vi "Label Printing.vi"(6 "Print?":bool, 7 "PN":string, 8 "error in (no error)":errorcluster, 9 "SN":string, 10 "DT":string, 11 "Path":path=path "D:/Valeo/Micriphone Test/UI/ME79.btw") -> (0 "error out":errorcluster)   [LabVIEW 2018]
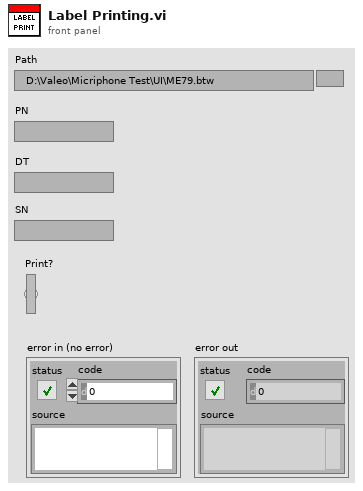
[diagram p1: front panel]
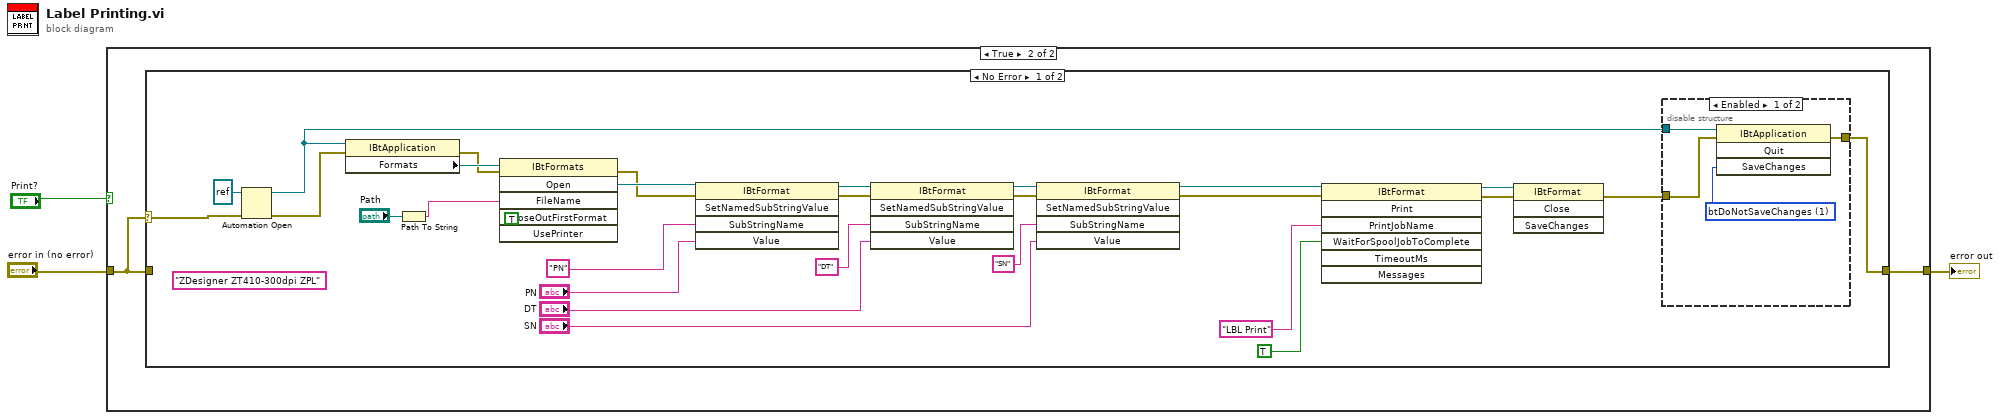
[diagram p0: block diagram]
diagram:
  n1 = case shown="True" "Print?" {
    tunnel: "error in (no error)" -> [w4 w5]
    tunnel: [w4 w6] -> w1
    frame False {
    }
    frame True {
      n2 = case shown="No Error" w5 {
        selector: w5 -> [w26 _]
        tunnel: [w27 w40] -> w6
        tunnel: w5 -> [_ w40]
        frame No Error {
          (unwired) "ZDesigner ZT410-300dpi ZPL" ("UsePrinter")
          (unwired) TRUE ("CloseOutFirstFormat")
          n3 = Automation Open(error in (no error)=w26, Automation Refnum=refnum<k7> refnum ("BarTender.IBtApplication")) -> (Automation Refnum=w13:refnum<k7>, error out=w12:errorcluster)  [unwired: 2 in]
          n4 = property class="IBtApplication"(reference=w13, error in=w12) -> (error out=w8:errorcluster, "Formats"=w11:refnum<k7>)  [unwired: 1 out]
          n5 = Path To String(path="Path") -> (string=w9:string)
          n6 = invoke class="IBtFormats" method="Open"(reference=w11, error in=w8, "FileName"=w9) -> (error out=w7:errorcluster, "Open"=w10:refnum<k7>)  [unwired: 3 in, 4 out]
          n7 = invoke class="IBtFormat" method="SetNamedSubStringValue"(reference=w10, error in=w7, "SubStringName"="PN" ("FieldnameSampleDataList"), "Value"="PN") -> (reference out=w25:refnum<k7>, error out=w22:errorcluster)  [unwired: 1 in, 3 out]
          n8 = invoke class="IBtFormat" method="SetNamedSubStringValue"(reference=w25, error in=w22, "SubStringName"="DT" ("FieldnameSampleDataList"), "Value"="DT") -> (reference out=w24:refnum<k7>, error out=w21:errorcluster)  [unwired: 1 in, 3 out]
          n9 = invoke class="IBtFormat" method="SetNamedSubStringValue"(reference=w24, error in=w21, "SubStringName"="SN" ("FieldnameSampleDataList"), "Value"="SN") -> (reference out=w23:refnum<k7>, error out=w20:errorcluster)  [unwired: 1 in, 3 out]
          n10 = invoke class="IBtFormat" method="Print"(reference=w23, error in=w20, "PrintJobName"="LBL Print", "WaitForSpoolJobToComplete"=TRUE) -> (reference out=w32:refnum<k7>, error out=w31:errorcluster)  [unwired: 3 in, 5 out]
          n11 = invoke class="IBtFormat" method="Close"(reference=w32, error in=w31) -> (error out=w30:errorcluster)  [unwired: 2 in, 3 out]
          n12 = disable-structure shown="Enabled" {
            disable-tunnel: w30 -> [w37 w39]
            disable-tunnel: [w36 w39] -> w27
            disable-tunnel: w13 -> [w35 _]
            frame Enabled {
              w38 = 1 items=["btPromptSave", "btDoNotSaveChanges", "btSaveChanges"] ("SaveChanges")
              n13 = invoke class="IBtApplication" method="Quit"(reference=w35, error in=w37, "SaveChanges"=w38) -> (error out=w36:errorcluster)  [unwired: 1 in, 3 out]
            }
            frame Disabled {
            }
          }
        }
        frame Error {
        }
      }
    }
  }
  "error out" <- w1
